vi "Dashboard Main.vi"() -> ()   [LabVIEW 2018]
uses:
  <vilib>/Utility/miscctls.llb/LVRowAndColumnTypeDef.ctl
  <vilib>/event_ctls.llb/eventvkey.ctl
  <vilib>/Rock Robotics/Network Tables/NT Read Numeric Array.vi
  <vilib>/Rock Robotics/WPI/Dashboard/WPI_DashboardLogging Global.vi
panel:
  in  "Camera Settings Right":T1={"Frame Rate"=30, "Compression"=30, "Size"=1, "DB Camera Config"=FALSE} {"Frame Rate" scale=1.0..30.0; "Compression" scale=100.0..-1.0; "Size" items=["640x480", "320x240", "160x120"]}
  in  "Camera Name Right":string(combo)="No Camera Selection"
  out "Camera Perf":string
  in  "Camera Settings":T1={"Frame Rate"=30, "Compression"=30, "Size"=1, "DB Camera Config"=FALSE} {"Frame Rate" scale=1.0..30.0; "Compression" scale=100.0..-1.0; "Size" items=["640x480", "320x240", "160x120"]}
  in  "TCP":refnum<k5>
  in  "Rec Mode":enum32{"Stop", "Record", "Playback"}(radio)
  out "Robot IP":string
  out "Image Message":string="Timeout in Camera Communications"
  in  "Dashboard Tab":T2(tab)
  out "Distance":dbl
  out "y2 (R)":dbl
  out "x2 (R)":dbl
  out "y1 (L)":dbl
  out "x1 (L)":dbl
  in  ".Avg Factor":i32=1
  in  "Enable Vision\nProcessing":bool
  in  "Reset":bool
  out "Total Stored\nSince Reset":i32
  in  "# New Images\nto Store":i32=1
  in  "Photo\nStore Rate":u32=100
  in  "Start\nStoring":bool
  in  "Select Auto":string(combo)="Select Autonomous ..."
  out "NT Connection":bool
  out "MotorChart R":cluster{"Numeric":dbl, "Numeric":dbl}(graph)
  out "MotorChart L":cluster{"Numeric":dbl, "Numeric":dbl}(graph)
  out "MotorSliders R":cluster{"MotorSlide1":dbl, "MotorSlide2":dbl} {"MotorSlide2" scale=-1.0..1.0 scale format="%#_2e"; "MotorSlide1" scale=-1.0..1.0 scale format="%#_2e"}
  out "MotorSliders L":cluster{"MotorSlide1":dbl, "MotorSlide2":dbl} {"MotorSlide2" scale=-1.0..1.0 scale format="%#_2e"; "MotorSlide1" scale=-1.0..1.0 scale format="%#_2e"}
  out "Gyro":dbl(knob) scale=0.0..360.0
  out "JS1 Z":dbl(slide) scale=-1.0..1.0 scale format="%#_2e"
  out "JS1 Graph":cluster{"X":dbl, "Y":dbl}[](graph)
  out "JS1 Buttons":T3
  out "JS2 Z":dbl(slide) scale=-1.0..1.0 scale format="%#_2e"
  out "JS2 Graph":cluster{"X":dbl, "Y":dbl}[](graph)
  out "JS2 Buttons":T3
  out "Mode":T4(ring)=enum."Auto Disabled"
  out "Right Camera Perf":cluster{"Bandwidth (Mbps)":dbl, "FPS":dbl}
  out "Camera Image Right":T5(plugin-control)
  in  "DB/String 9":string
  in  "DB/String 8":string
  in  "DB/String 7":string
  in  "DB/String 6":string
  in  "DB/String 5":string
  in  "DB/String 4":string
  in  "DB/String 3":string
  in  "DB/String 2":string
  in  "DB/String 1":string
  in  "DB/String 0":string
  in  "DB/Slider 0":dbl(slide) scale=0.0..5.0
  in  "DB/Slider 1":dbl(slide) scale=0.0..5.0
  in  "DB/Slider 2":dbl(slide) scale=0.0..5.0
  in  "DB/Slider 3":dbl(slide) scale=0.0..5.0
  out "DB/LED 3":bool
  out "DB/LED 2":bool
  out "DB/LED 1":bool
  out "DB/LED 0":bool
  in  "DB/Button 3":bool
  in  "DB/Button 2":bool
  in  "DB/Button 1":bool
  in  "DB/Button 0":bool caption="New Name"
  in  "Test Slider":dbl(slide) scale=0.0..100.0 scale format="%#_3g"
  in  "On/Off":bool caption="Solenoid"
  in  "Test Name":u16(ring) items=["Select the test to run..."]
  in  "Test Tree":string(tree)
  in  "Motor":cluster{"Value":dbl, "Enable":bool} {"Value" scale=-1.0..1.0 scale format="%#_3g"}
  out "Progress":T6 {"Test Progress" scale=0.0..100.0}
  in  "Rev/Fwd":cluster{"Forward":bool, "Reverse":bool}
  in  "Test Ring":u16(ring) items=["Monochrome", "Color"]
  out "Cmd Status":string
  in  "Execute Command":bool
  in  "Command Params":string[][](table)
  in  "Command Selection":i32(listbox)
  in  "CheckList":i32(listbox)
  out "Tree":string(tree)
  out "Camera Image":T5(plugin-control)
  out "Background":bool
  in  "Camera Name":string(combo)="No Camera Selection"
  # "HW"
  # "HW"
  # "Joysticks"
  # "Drive Motors"
  # "Front"
  # "Right"
  # "Left"
  # "Back"
  # "This tab is a great place for autonomous settings and robot-specific values.\nPlace controls and indicators inside this tab and match name to\nDashboard Variables on robot. You can also delete this comment."
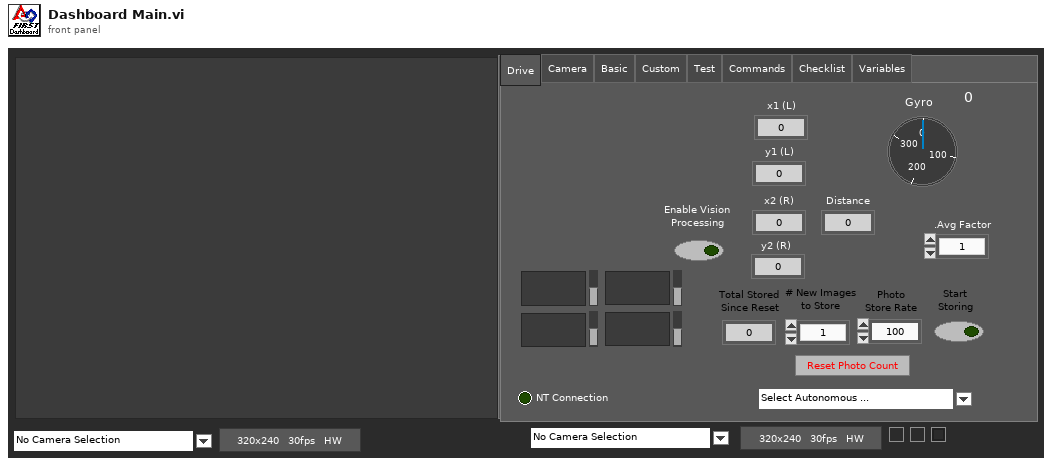
[diagram p1: front panel]
types:
  T1 = cluster{"Frame Rate":i32, "Compression":i32, "Size":u16, "DB Camera Config":bool}
  T2 = enum32{"Drive", "Camera", "Basic", "Custom", "Test", "Commands", "Checklist", "Variables"}
  T3 = cluster{bool, bool, bool, bool, bool, bool, bool, bool, bool, bool, bool, bool}
  T4 = enum8{"Tele-Op Disabled", "Tele-Op Enabled", "Auto Disabled", "Auto Enabled", "Test Disabled", "Test Enabled", "Disconnected", "No Code", "E-Stop"}
  T5 = typedef "IMAQ Image.ctl" = refnum<image>
  T6 = cluster{"Test Progress":u8, "Test Progress Text":string}
  T7 = cluster{"Save Path":path, "Interval (s)":dbl, "Keep":i32}
  T8 = typedef "Image Type" = u32
  T9 = cluster{"IDs":cluster{"RPC field ID":u16, "Unique ID":u16}, "String":string}
  T10 = cluster{"Camera Image":refnum<vi>, "Dashboard Tab":refnum<vi>, "Background":refnum<vi>, "Rec Mode":refnum<vi>, "Test Slider":refnum<vi>, "On/Off ":refnum<vi>, "Test Ring":refnum<vi>, "Rev/Fwd":refnum<vi>, "Test Name":refnum<vi>, "Motor":refnum<vi>, "Progress":refnum<vi>, "CheckList":refnum<vi>, "Tree":refnum<vi>, "Test Tree":refnum<vi>, "Command Params":refnum<vi>, "Command Selection":refnum<vi>, "Execute Command":refnum<vi>, "Cmd Status":refnum<vi>, "Camera Settings":refnum<vi>, "Camera Name":refnum<vi>, "Camera Perf":refnum<vi>, "Camera Settings Right":refnum<vi>, "Camera Name Right":refnum<vi>, "Camera Image Right":refnum<vi>}
  T11 = cluster{"Global Rectangle":i32[], "Contours":cluster{"Contour Type":u32, "ROI Type":u32, "Points":i32[]}[]}
  T12 = cluster{"Camera Name":string, string, "Saved DB Images Info":cluster{"Save Path":path, "Interval (s)":dbl, "Keep":i32}}
  T13 = cluster{"Pixels ":cluster{"Start":cluster{"X":dbl, "Y":dbl}, "End":cluster{"X":dbl, "Y":dbl}}, "Real World":cluster{"Start":cluster{"X":dbl, "Y":dbl}, "End":cluster{"X":dbl, "Y":dbl}}}
  T14 = cluster{"Start":cluster{"X":dbl, "Y":dbl}, "End":cluster{"X":dbl, "Y":dbl}}
  T15 = cluster{"Camera Name Right":string, string, "Saved DB Images Info":cluster{"Save Path":path, "Interval (s)":dbl, "Keep":i32}}
  T16 = cluster{"Error Strings":string, "Disable Counts":cluster{u16, u16}, "Rail Faults":cluster{u16, u16, u16}, "Robot IP":string, "DB Mode":u8, "Event Info":cluster{"Name":string, "Type":u8, "Number":u16, "Replay":u8}}
  T17 = cluster{"Storage":cluster{"Disk Free":u64, "RAM Block":u32, "RAM free":u32}, "CPU Utilization":cluster{"CPU % ISR":sgl, "CPU % Time Crit":sgl, "CPU % Timed Str":sgl, "CPU % High":sgl, "CPU % Above":sgl, "CPU % Normal":sgl, "CPU % Low":sgl}, "CAN":cluster{"% Bus Utilization":sgl, "Bus Off Cnt":u32, "TX_FIFO Full Cnt":u32, "Receive Error Cnt":u8, "Transmit Error Cnt":u8}, "HID":cluster{"HID Outputs":u32, "Rumble Low":u16, "Rumble High":u16}[]}
  T18 = cluster{"Status bits":cluster{"Test Mode":bool, "Autonomous":bool, "Enabled":bool, "Code Start":bool, "Brownout":bool, "Reserved 2":bool, "Reserved 3":bool, "E-Stop":bool}, "Code Trace":cluster{"Disabled":bool, "TeleOp":bool, "Auto":bool, "Test":bool}, "Controller Type":enum16{"unknown", "cRIO", "roboRio"}, "Code?":enum16{"unknown", "noCode", "code"}, "Battery V":dbl}
  T19 = cluster{"Control Bits":cluster{"TestMode":bool, "Autonomous":bool, "Enabled":bool, "FMS Present":bool, bool, bool, bool, "E-Stop":bool}, "Team Station ":u8, "Countdown":sgl, "Joystick Values":cluster{"Axes":dbl[], "Buttons":bool[], "POVs":i16[]}[]}
  T20 = cluster{"Axes":dbl[], "Buttons":bool[], "POVs":i16[]}[]
  T21 = cluster{"Axes":dbl[], "Buttons":bool[], "POVs":i16[]}
  T22 = cluster{"Buttons[0]":bool, "Buttons[1]":bool, "Buttons[2]":bool, "Buttons[3]":bool, "Buttons[4]":bool, "Buttons[5]":bool, "Buttons[6]":bool, "Buttons[7]":bool, "Buttons[8]":bool, "Buttons[9]":bool, "Buttons[10]":bool, "Buttons[11]":bool}
  T23 = cluster{"Operation":enum16{"Update", "Clear"}, "Color Box":u32}[]
  T24 = typedef "eventvkey.ctl" = enum16{"ASCII", "Enter", "Return", "Shift", "Ctrl", "Alt", "Cmd", "Opt", "Caps", "NumLock", "Clear", "Break", "Up", "Down", "Left", "Right", "Insert", "Delete", "Home", "End", "PageUp", "PageDown", "Escape", "Help", "Pause", "ScrollLock", "F1", "F2", "F3", "F4", "F5", "F6", "F7", "F8", "F9", "F10", "F11", "F12", "F13", "F14", "F15", "F16", "F17", "F18", "F19", "F20", "F21", "F22", "F23", "F24", "Play", "VolumeUp", "VolumeDown", "Mute", "Two Byte Char"}
  T25 = cluster{"Image Size":bool, "Image Type":bool, "Pixel Value":bool, "ROI Information":bool, "Zoom Factor":bool}
  T26 = cluster{"Operation":enum16{"Update", "Clear"}, "Color Box":u32}
  T27 = typedef "LVRowAndColumnTypeDef.ctl" = cluster{"Row":i32, "Column":i32}
  T28 = cluster{"Shift":bool, "Ctrl":bool, "Alt":bool, "Cmd":bool, "Opt":bool}
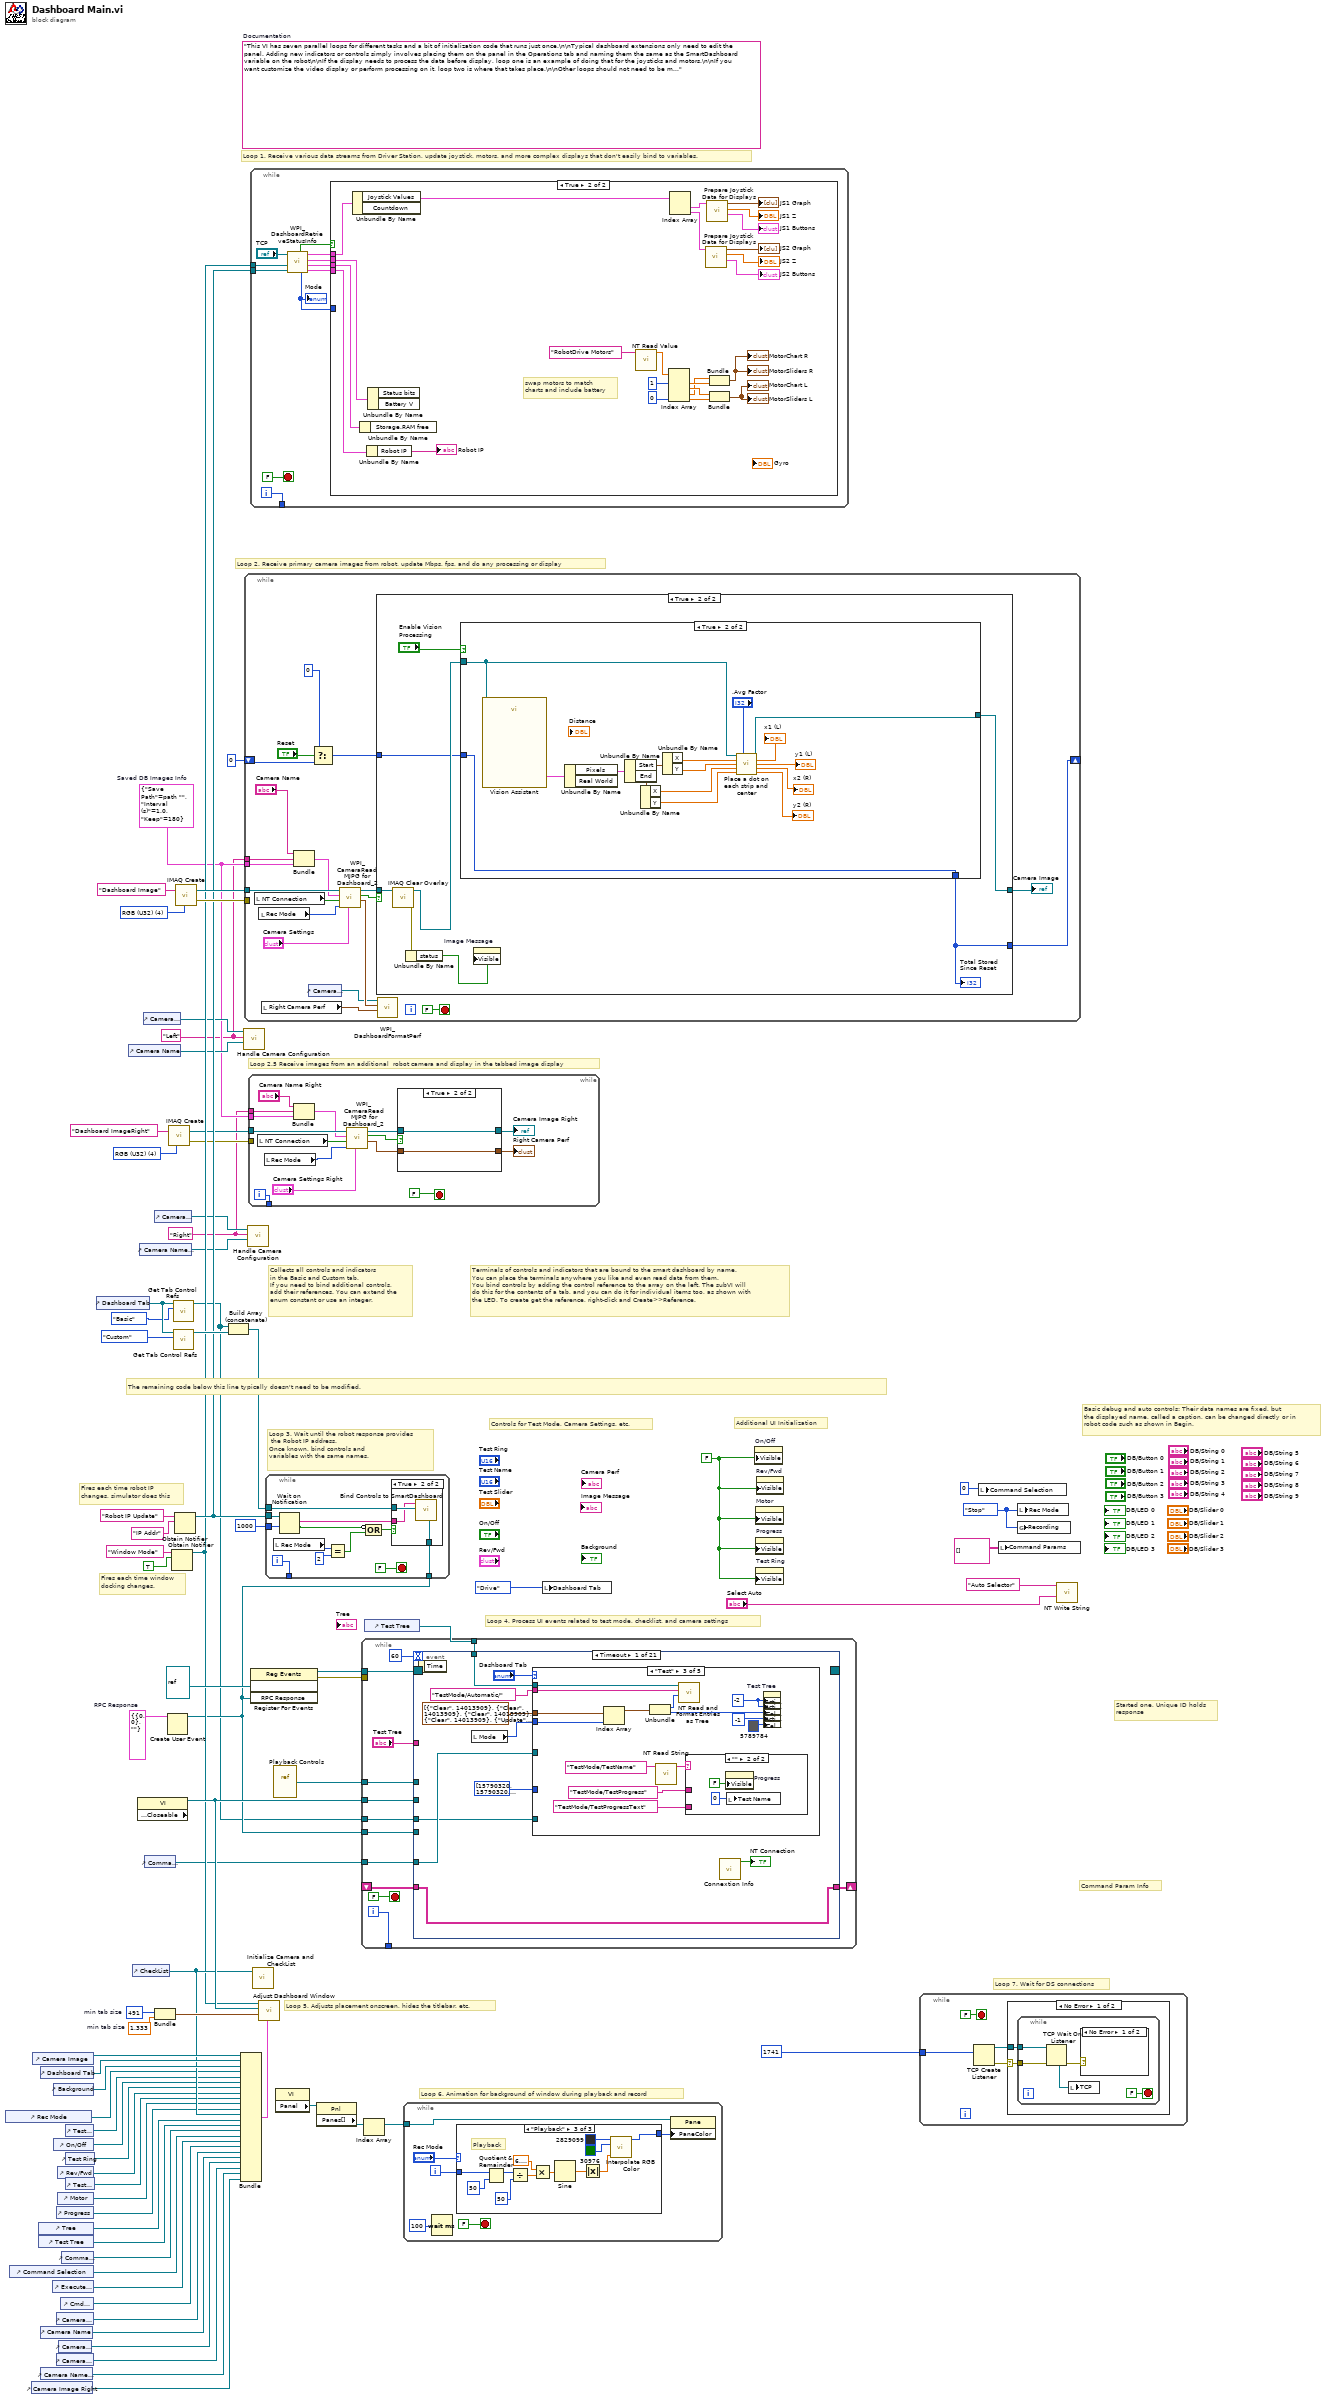
[diagram p0: block diagram]
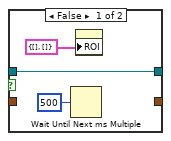
[diagram p2: hidden frame]
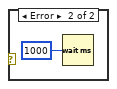
[diagram p3: hidden frame]
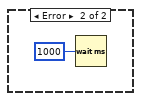
[diagram p4: hidden frame]
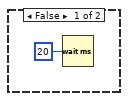
[diagram p5: hidden frame]
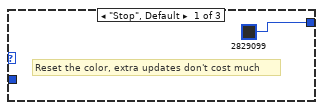
[diagram p6: hidden frame]
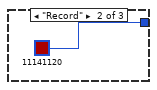
[diagram p7: hidden frame]
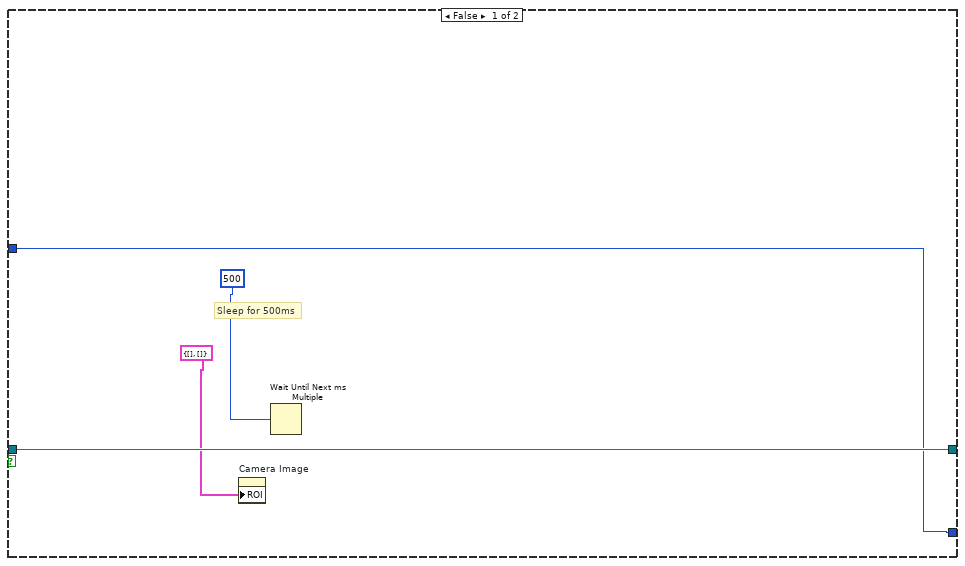
[diagram p9: hidden frame]
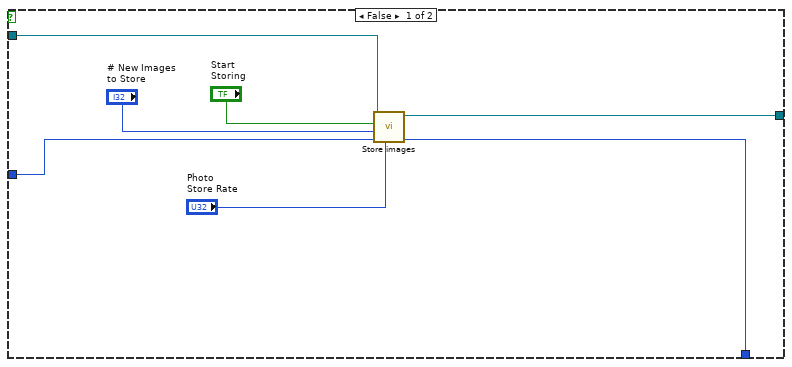
[diagram p10: hidden frame]
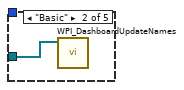
[diagram p12: hidden frame]
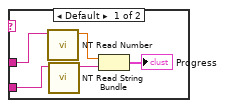
[diagram p13: hidden frame]
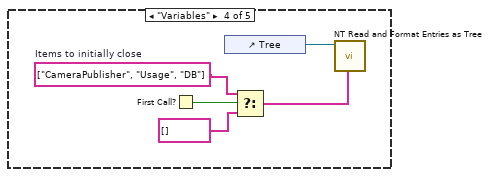
[diagram p14: hidden frame]
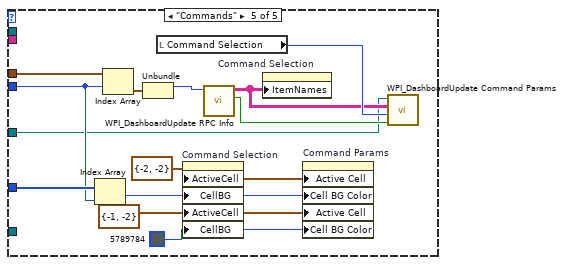
[diagram p15: hidden frame]
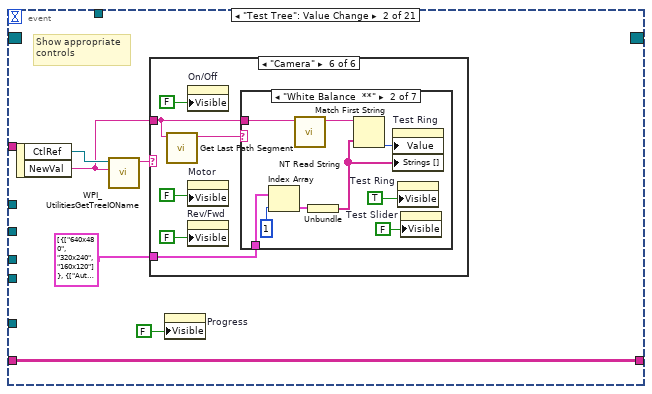
[diagram p16: hidden frame]
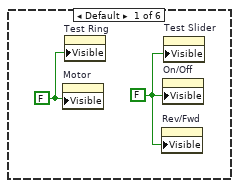
[diagram p17: hidden frame]
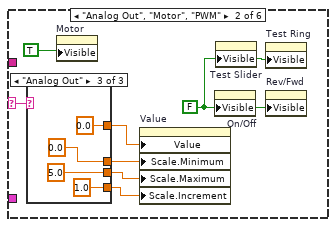
[diagram p18: hidden frame]
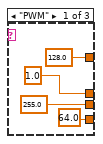
[diagram p19: hidden frame]
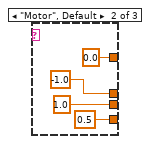
[diagram p20: hidden frame]
diagram:
  w4 = T7 {"Save Path"=path "", "Interval (s)"=1.0, "Keep"=180}  # Saved DB Images Info
  w3 = "Right"
  w2 = "Left"
  w14 = T8 4 items=["Grayscale (U8)", "Grayscale (I16)", "Grayscale (SGL)", "Complex (CSG)", "RGB (U32)", "HSL (U32)", "RGB (U64)"] ("Image Type")
  w30 = T9 {"IDs"={"RPC field ID"=0, "Unique ID"=0}, "String"=""}  # RPC Response
  w53 = 491  # min tab size
  w52 = 1.333  # min tab size
  w60 = enum32{"Stop", "Record", "Playback"}."Stop" ("Rec Mode")
  w37 = FALSE ("Visible")
  (unwired) "This VI has seven parallel loops for different tasks and a bit of initialization code that runs just once.\n\nTypical dashboard extensions only need to edit the panel. Adding new indicators or controls simply involves placing them on the panel in the Operations tab and naming them the same as the SmartDashboard variable on the robot\n\nIf the display needs to process the data before display, loop one is an example of doing that for the joysticks and motors.\n\nIf you want customize the video display or perform processing on it, loop two is where that takes place.\n\nOther loops should not need to be modified. They are pretty standard, and document the task they perform."  # Documentation
  w77 = T8 4 items=["Grayscale (U8)", "Grayscale (I16)", "Grayscale (SGL)", "Complex (CSG)", "RGB (U32)", "HSL (U32)", "RGB (U64)"] ("Image Type")
  # "Loop 2.5 Receive images from an additional  robot camera and display in the tabbed image display"
  # "Command Param Info"
  # "Started one, Unique ID holds\nresponse"
  # "Loop 7. Wait for DS connections"
  # "Basic debug and auto controls: Their data names are fixed, but\nthe displayed name, called a caption, can be changed directly or in\nrobot code such as shown in Begin."
  # "Controls for Test Mode, Camera Settings, etc."
  # "Additional UI Initialization"
  # "Loop 6. Animation for background of window during playback and record"
  # "Fires each time robot IP\nchanges, simulator does this"
  # "Fires each time window\ndocking changes."
  # "Collects all controls and indicators\nin the Basic and Custom tab.\nIf you need to bind additional controls,\nadd their references. You can extend the\nenum constant or use an integer."
  # "The remaining code below this line typically doesn't need to be modified."
  # "Loop 4. Process UI events related to test mode, checklist, and camera settings"
  # "Terminals of controls and indicators that are bound to the smart dashboard by name.\nYou can place the terminals anywhere you like and even read data from them.\nYou bind controls by adding the control reference to the array on the left. The subVI will\ndo this for the contents of a tab, and you can do it for individual items too, as shown with\nthe LED. To create get the reference, right-click and Create>>Reference."
  # "Loop 3. Wait until the robot response provides\n the Robot IP address.\nOnce known, bind controls and\nvariables with the same names."
  # "Loop 5. Adjusts placement onscreen, hides the titlebar, etc."
  # "Loop 1. Receive various data streams from Driver Station, update joystick, motors, and more complex displays that don't easily bind to variables."
  # "Loop 2. Receive primary camera images from robot, update Mbps, fps, and do any processing or display"
  n1 = control-ref of="Rec Mode"() -> (w43:refnum<vi>)
  n2 = control-ref of="Command Selection"() -> (w29:refnum<vi>)
  n3 = control-ref of="Camera Image Right"() -> (w7:refnum<vi>)
  n4 = control-ref of="Camera Image"() -> (w55:refnum<vi>)
  n5 = control-ref of="Tree"() -> (w47:refnum<vi>)
  n6 = control-ref of="Test Tree"() -> (w46:refnum<vi>)
  n7 = control-ref of="Dashboard Tab"() -> (w54:refnum<vi>)
  n8 = control-ref of="Camera Name"() -> (w20:refnum<vi>)
  n9 = control-ref of="Camera Name Right"() -> (w8:refnum<vi>)
  n10 = control-ref of="Execute Command"() -> (w31:refnum<vi>)
  n11 = control-ref of="Background"() -> (w50:refnum<vi>)
  n12 = control-ref of="On/Off"() -> (w41:refnum<vi>)
  n13 = control-ref of="Progress"() -> (w38:refnum<vi>)
  n14 = control-ref of="Camera Settings"() -> (w21:refnum<vi>)
  n15 = control-ref of="Camera Settings Right"() -> (w9:refnum<vi>)
  n16 = control-ref of="Rev/Fwd"() -> (w39:refnum<vi>)
  n17 = control-ref of="Motor"() -> (w44:refnum<vi>)
  n18 = control-ref of="Camera Perf"() -> (w19:refnum<vi>)
  n19 = control-ref of="Cmd Status"() -> (w25:refnum<vi>)
  n20 = control-ref of="Command Params"() -> (w32:refnum<vi>)
  n21 = control-ref of="Test Slider"() -> (w42:refnum<vi>)
  n22 = control-ref of="Test Ring"() -> (w40:refnum<vi>)
  n23 = control-ref of="Test Name"() -> (w45:refnum<vi>)
  n24 = control-ref of="Dashboard Tab"() -> (w58:refnum<vi>)
  n25 = control-ref of="Camera Name"() -> (w22:refnum<vi>)
  n26 = control-ref of="CheckList"() -> (w48:refnum<vi>)
  n27 = property class="VI" props=["Front Panel.Closeable"]() -> (reference out=w59:refnum<vi>)  [unwired: 2 in, 2 out]
  n28 = control-ref of="Camera Name Right"() -> (w10:refnum<vi>)
  n29 = control-ref of="Camera Settings"() -> (w23:refnum<vi>)
  n30 = control-ref of="Command Params"() -> (w24:refnum<vi>)
  n31 = control-ref of="Camera Settings Right"() -> (w11:refnum<vi>)
  n32 = Bundle("min tab size"=w53, "min tab size"=w52) -> (w51:cluster{"min tab size":i32, "min tab size":dbl})  [unwired: 1 in]
  n33 = Create User Event(user event datatype=w30) -> (user event=w26:refnum<user-event>)  [unwired: 1 in, 1 out]
  n34 = call "IMAQ Create"("Image Name"="Dashboard ImageRight", "Image Type"=w14) -> ("New Image"=w13:T5, "error out"=w12:errorcluster)  [unwired: 2 in, 1 out]
  n35 = Obtain Notifier(name (unnamed)="Window Mode", notification data type=TRUE) -> (notifier out=w35:refnum<notifier>)  [unwired: 2 in, 2 out]
  n36 = call <vilib>:"Get Tab Control Refs.vi"("Page Index"=T2."Basic" ("Dashboard Tab"), "TabControl in"=w58) -> ("ControlsOnPage"=w18:refnum<vi>[])  [unwired: 9 in]
  n37 = call <vilib>:"Get Tab Control Refs.vi"("Page Index"=T2."Custom" ("Dashboard Tab"), "TabControl in"=w58) -> ("ControlsOnPage"=w57:refnum<vi>[])  [unwired: 9 in]
  n38 = Obtain Notifier(name (unnamed)="Robot IP Update", notification data type="IP Addr" ("name (unnamed)")) -> (notifier out=w36:refnum<notifier>)  [unwired: 2 in, 2 out]
  n39 = call "IMAQ Create"("Image Name"="Dashboard Image", "Image Type"=w77) -> ("New Image"=w75:T5, "error out"=w74:errorcluster)  [unwired: 2 in, 1 out]
  n40 = Build Array (concatenate)(w18, w57) -> (w56:refnum<vi>[])
  n41 = Bundle("Camera Image"=w55, "Dashboard Tab"=w54, "Background"=w50, "Rec Mode"=w43, "Test Slider"=w42, "On/Off"=w41, "Test Ring"=w40, "Rev/Fwd"=w39, "Test Name"=w45, "Motor"=w44, "Progress"=w38, "CheckList"=w48, "Tree"=w47, "Test Tree"=w46, "Command Params"=w32, "Command Selection"=w29, "Execute Command"=w31, "Cmd Status"=w25, "Camera Settings"=w21, "Camera Name"=w20, "Camera Perf"=w19, "Camera Settings Right"=w9, "Camera Name Right"=w8, "Camera Image Right"=w7) -> (w49:T10)  [unwired: 1 in]
  n42 = call "Handle Camera Configuration.vi"("CameraNameRef"=w22, "Display Name"=w2, "ClusterRef"=w23) -> ()  [unwired: 9 in]
  n43 = while {
    tunnel: w75 -> [w96]
    tunnel: w74 -> [_]
    tunnel: w4 -> [w89]
    tunnel: w2 -> [w86]
    shift-right: [w78] -> _
    shift-left: 0 -> [w81]
    stop <- FALSE stop-if-true
    n44 = local read "NT Connection"() -> (w90:bool)
    n45 = local read "Rec Mode"() -> (w93:enum32{"Stop", "Record", "Playback"})
    n46 = local read "Right Camera Perf"() -> (w84:cluster{"Bandwidth (Mbps)":dbl, "FPS":dbl})
    n47 = Bundle("Camera Name"="Camera Name", w86, "Saved DB Images Info"=w89) -> (w88:T12)  [unwired: 1 in]
    n48 = control-ref of="Camera Perf"() -> (w83:refnum<vi>)
    n49 = Select(t=0, s="Reset", f=w81) -> (s? t:f=w79:i32)
    n50 = call <vilib>:"WPI_CameraRead MJPG for Dashboard_2.vi"("Camera Settings"="Camera Settings", "Rec Mode"=w93, "NT Connection"=w90, "Capture Info"=w88, "Image in"=w96) -> ("perf info"=w85:cluster{"Bandwidth (Mbps)":dbl, "fps":dbl}, "Active"=w94:bool, "Image\\ out"=w95:T5)  [unwired: 4 in]
    n51 = case shown="True" w94 {
      tunnel: w95 -> [w100 w107]
      tunnel: [w100 w103] -> w91
      tunnel: w79 -> [w98 w104]
      tunnel: [w98 w102] -> w78
      frame False {
        # "Sleep for 500ms"
        n52 = property on="Camera Image" class="ImageControl"("ROI"=T11 {"Global Rectangle"=[], "Contours"=[]}) -> ()  [unwired: 2 in, 2 out]
        n53 = Wait Until Next ms Multiple(millisecond multiple=u32 500) -> ()  [unwired: 1 out]
      }
      frame True {
        n54 = call "IMAQ Clear Overlay"("Image"=w107) -> ("error out"=w108:errorcluster, "Image Out"=w105:T5)  [unwired: 2 in, 7 out]
        n55 = Unbundle By Name(w108) -> ("status"=w109:bool)
        n56 = case shown="True" "Enable Vision\nProcessing" {
          tunnel: w105 -> [w113 w124]
          tunnel: w104 -> [w112 w130]
          tunnel: [w111 w123] -> w103
          tunnel: [w110 w130] -> w102
          frame False {
            n57 = call "Store images.vi"("ms Capture Rate"="Photo\nStore Rate", "# Total images IN"=w112, "# new images to capture"="# New Images\nto Store", "Store # Images?"="Start\nStoring", "Image"=w113) -> ("Total images OUT"=w110:i32, "Image Out"=w111:T5)  [unwired: 5 in]
          }
          frame True {
            n58 = call "Vision Assistant"("Image In"=w124) -> ("Clamp Points (Max Clamp 1)"=w132:T13)  [unwired: 23 in, 3 out]
            n59 = Unbundle By Name(w132) -> ("Pixels"=w131:T14)  [unwired: 1 out]
            n60 = Unbundle By Name(w131) -> ("Start"=w129:cluster{"X":dbl, "Y":dbl}, "End"=w128:cluster{"X":dbl, "Y":dbl})
            n61 = Unbundle By Name(w128) -> ("X"=w118:dbl, "Y"=w117:dbl)
            n62 = Unbundle By Name(w129) -> ("X"=w127:dbl, "Y"=w126:dbl)
            n63 = call "Place a dot on each strip and center.vi"("Image"=w124, "Avg Factor"=".Avg Factor", "x1 (L) IN"=w127, "y1 (L) IN"=w126, "x2 (R) IN"=w118, "y2 (R) IN"=w117) -> ("Image Out"=w123:T5, "x1 (L) out"=→"x1 (L)":dbl, "y1 (L) out"=→"y1 (L)":dbl, "x2 (R) out"=→"x2 (R)":dbl, "y2 (R) out"=→"y2 (R)":dbl)  [unwired: 5 in]
          }
        }
        "Total Stored\nSince Reset" <- w102
        n64 = property on="Image Message" class="Str"("Visible"=w109) -> ()  [unwired: 2 in, 2 out]
      }
    }
    "Camera Image" <- w91
    n65 = call <vilib>:"WPI_DashboardFormatPerf.vi"("Right Camera Perf"=w84, "Performance"=w85, "String in"=w83) -> ()  [unwired: 9 in]
  }
  n66 = call "Handle Camera Configuration.vi"("CameraNameRef"=w10, "Display Name"=w3, "ClusterRef"=w11) -> ()  [unwired: 9 in]
  n67 = while {
    tunnel: w13 -> [w147]
    tunnel: w12 -> [_]
    tunnel: [w142] -> _
    tunnel: w4 -> [w138]
    tunnel: w3 -> [w135]
    i -> [w142]
    stop <- FALSE stop-if-true
    n68 = local read "NT Connection"() -> (w139:bool)
    n69 = local read "Rec Mode"() -> (w146:enum32{"Stop", "Record", "Playback"})
    n70 = Bundle("Camera Name Right"="Camera Name Right", w135, "Saved DB Images Info"=w138) -> (w137:T15)  [unwired: 1 in]
    n71 = call <vilib>:"WPI_CameraRead MJPG for Dashboard_2.vi"("Camera Settings"="Camera Settings Right", "Rec Mode"=w146, "NT Connection"=w139, "Capture Info"=w137, "Image in"=w147) -> ("perf info"=w133:cluster{"Bandwidth (Mbps)":dbl, "fps":dbl}, "Active"=w141:bool, "Image\\ out"=w144:T5)  [unwired: 4 in]
    n72 = case shown="True" w141 {
      tunnel: w144 -> [w149 w152]
      tunnel: [w149 w152] -> w140
      tunnel: [_ w151] -> w134
      tunnel: w133 -> [_ w151]
      frame False {
        n73 = Wait Until Next ms Multiple(millisecond multiple=u32 500) -> ()  [unwired: 1 out]
        n74 = property on="Camera Image Right" class="ImageControl"("ROI"=T11 {"Global Rectangle"=[], "Contours"=[]}) -> ()  [unwired: 2 in, 2 out]
      }
      frame True {
      }
    }
    "Camera Image Right" <- w140
    "Right Camera Perf" <- w134
  }
  n75 = while {
    tunnel: [w162] -> _
    tunnel: w36 -> [w156]
    tunnel: w35 -> [w153]
    i -> [w162]
    stop <- FALSE stop-if-true
    n76 = call <vilib>:"WPI_DashboardRetrieveStatusInfo.vi"("Binding Refnum"=w156, "Window Mode Notifier"=w153, "TCP Cnx"="TCP") -> ("Power and Errors"=w157:T16, "Robot Metrics"=w160:T17, "Status Info"=w161:T18, "Control Info"=w158:T19, "Robot Mode"=w155:T4, "Process?"=w159:bool)  [unwired: 3 in]
    "Mode" <- w155
    n77 = case shown="True" w159 {
      tunnel: w161 -> [_ w188]
      tunnel: w160 -> [_ w187]
      tunnel: w158 -> [_ w186]
      tunnel: w157 -> [_ w185]
      tunnel: w155 -> [_ _]
      frame False {
        n78 = Wait (ms)(milliseconds to wait=u32 20) -> ()  [unwired: 1 out]
      }
      frame True {
        # "swap motors to match\ncharts and include battery"
        n79 = Unbundle By Name(w186) -> ("Joystick Values"=w176:T20)  [unwired: 1 out]
        n80 = Unbundle By Name(w187) -> ()  [unwired: 1 out]
        n81 = Unbundle By Name(w185) -> ("Robot IP"=→"Robot IP":string)
        n82 = Unbundle By Name(w188) -> ()  [unwired: 2 out]
        n83 = call-poly <vilib>:"NT Read Value.vi"("Name"="RobotDrive Motors") -> ("Numeric Array"=w166:dbl[])  [unwired: 9 in, 1 out]
        n84 = Index Array(array=w166, index #1=1, index #4=0) -> (element #1=w180:dbl, element #2=w181:dbl, element #3=w179:dbl, element #4=w184:dbl)  [unwired: 2 in]
        n85 = Index Array(array=w176) -> (element #1=w175:T21, element #2=w171:T21)  [unwired: 2 in]
        n86 = call "Prepare Joystick Data for Displays.vi"("Joystick Values"=w171) -> ("Buttons"=→"JS2 Buttons":T22, "Z Axis"=→"JS2 Z":dbl, "Cartesian Data"=→"JS2 Graph":cluster{"X axis":dbl, "X axis":dbl}[])  [unwired: 8 in]
        n87 = call "Prepare Joystick Data for Displays.vi"("Joystick Values"=w175) -> ("Buttons"=→"JS1 Buttons":T22, "Z Axis"=→"JS1 Z":dbl, "Cartesian Data"=→"JS1 Graph":cluster{"X axis":dbl, "X axis":dbl}[])  [unwired: 8 in]
        n88 = Bundle("Numeric"=w179, "Numeric"=w180) -> (→"MotorChart R" →"MotorSliders R":cluster{"Numeric":dbl, "Numeric":dbl})  [unwired: 1 in]
        n89 = Bundle("Numeric"=w181, "Numeric"=w184) -> (→"MotorChart L" →"MotorSliders L":cluster{"Numeric":dbl, "Numeric":dbl})  [unwired: 1 in]
      }
    }
  }
  n90 = register-events(refnum<vi> refnum, w26) -> (reference out=w64:refnum<event-registration>, error out=w63:errorcluster)  [unwired: 2 in]
  n91 = call "Initialize Camera and CheckList.vi"("ListBox in"=w48) -> ()  [unwired: 11 in]
  n92 = call "Adjust Dashboard Window.vi"("Sizing Refnums"=w49, "Size Constraints"=w51, "VI"=w59, "WIn Mode"=w35) -> ()  [unwired: 8 in]
  n93 = while {
    tunnel: w56 -> [w200]
    tunnel: w36 -> [w198]
    tunnel: [w196] -> _
    tunnel: u32 1000 ("milliseconds to wait") -> [w195]
    tunnel: w26 -> [w189]
    i -> [w196]
    stop <- FALSE stop-if-true
    n94 = local read "Rec Mode"() -> (w191:enum32{"Stop", "Record", "Playback"})
    n95 = Wait on Notification(notifier=w198, timeout in ms (-1)=w195) -> (notification=w197:string, timed out?=w193:bool)  [unwired: 2 in, 2 out]
    n96 = Equal?(x=w191, y=u16 2 ("Rec Mode")) -> (x = y?=w192:bool)
    n97 = Compound Arithmetic op=OR(invert w193, w192) -> (w194:bool)
    n98 = case shown="True" w194 {
      tunnel: w200 -> [_ w203]
      tunnel: w197 -> [_ w202]
      tunnel: w189 -> [_ w201]
      frame False {
      }
      frame True {
        n99 = call <vilib>:"Bind Controls to SmartDashboard.vi"("RPC ref"=w201, "Bound Control Refs"=w203, "Server IP Address"=w202) -> ()  [unwired: 9 in]
      }
    }
  }
  n100 = vi-ref "Playback Controls.vi"() -> (w65:refnum<vi>)
  n101 = property class="VI"() -> ("Panel"=w67:refnum<vi>)  [unwired: 2 in, 2 out]
  n102 = property class="Pnl"(reference=w67) -> ("Panes[]"=w68:refnum<vi>[])  [unwired: 1 in, 2 out]
  n103 = Index Array(array=w68) -> (element=w66:refnum<vi>)  [unwired: 1 in]
  n104 = control-ref of="Test Tree"() -> (w69:refnum<vi>)
  n105 = while {
    tunnel: [w213] -> _
    tunnel: w69 -> [w212]
    tunnel: w65 -> [w211]
    tunnel: w64 -> [w210]
    tunnel: w63 -> [_]
    tunnel: w59 -> [w209]
    tunnel: w26 -> [w208]
    tunnel: w24 -> [w207]
    shift-right: [w206] -> _
    shift-left: _ -> [w205]
    tunnel: w18 -> [w204]
    i -> [w213]
    stop <- FALSE stop-if-true
    n106 = event shown="[0] Timeout" {
      selector: w210 -> [_ _ _ _ _ _ _ _ _ _ _ _ _ _ _ _ _ _ _ _ _]
      dyn-events: [_ _ _ _ _ _ _ _ _ _ _ _ _ _ _ _ w473 _ _ _ _] -> _
      timeout: u32 60 ("milliseconds to wait") -> [_ _ _ _ _ _ _ _ _ _ _ _ _ _ _ _ _ _ _ _ _]
      tunnel: w212 -> [w225 _ _ _ _ _ _ _ _ _ _ _ _ _ _ _ _ _ _ _ _]
      tunnel: "Test Tree" -> [_ _ _ _ _ _ _ _ _ _ _ w440 w448 w450 w454 w462 _ _ _ _ _]
      tunnel: w211 -> [_ _ _ _ _ _ _ _ _ _ _ _ _ _ _ _ w475 _ w493 _ _]
      tunnel: w209 -> [_ _ _ _ _ _ _ _ _ _ _ _ _ _ _ _ w471 _ _ _ _]
      tunnel: w208 -> [_ _ _ _ _ _ _ _ _ _ _ _ _ _ _ _ w469 _ _ _ _]
      tunnel: w207 -> [w220 _ _ _ _ _ w391 _ _ _ _ _ _ _ _ _ _ _ _ _ _]
      tunnel: [w219 w268 w370 w375 w384 w388 w389 w398 w408 w415 w427 w439 w446 w449 w453 w461 w468 w488 w490 w494 w507] -> w206
      tunnel: w205 -> [w219 w268 w370 w375 w384 w388 w389 _ _ w415 w427 w439 w446 w449 w453 w461 w468 w488 w490 w494 w507]
      tunnel: w204 -> [w217 _ _ _ _ _ _ _ _ _ _ _ _ _ _ _ _ _ _ _ _]
      event Timeout {
        n107 = event-data() -> ()  [unwired: 1 in, 1 out]
        n108 = local read "Mode"() -> (w222:T4)
        n109 = case shown="\"Test\"" "Dashboard Tab" {
          tunnel: w225 -> [_ _ w241 _ _]
          tunnel: "TestMode/Automatic/" ("Name Pattern") -> [_ _ w240 _ _]
          tunnel: T23 [{"Operation"=enum."Clear", "Color Box"=14013909}, {"Operation"=enum."Clear", "Color Box"=14013909}, {"Operation"=enum."Clear", "Color Box"=14013909}, {"Operation"=enum."Clear", "Color Box"=14013909}, {"Operation"=enum."Update", "Color Box"=14013909}, {"Operation"=enum."Update", "Color Box"=16777215}, {"Operation"=enum."Clear", "Color Box"=14013909}, {"Operation"=enum."Clear", "Color Box"=14013909}, {"Operation"=enum."Clear", "Color Box"=14013909}] -> [_ _ w233 _ w261]
          tunnel: w222 -> [_ _ w232 _ w260]
          tunnel: u32[] [15790320, 15790320, 15790320, 15790320, 16777215, 16777215, 15790320, 15790320, 15790320] -> [_ _ _ _ w266]
          tunnel: w220 -> [_ _ _ _ w254]
          tunnel: w217 -> [_ w227 _ _ _]
          frame "Custom", Default {
          }
          frame "Basic" {
            n110 = call <vilib>:"WPI_DashboardUpdateNames.vi"("Controls on Tab"=w227) -> ()  [unwired: 11 in]
          }
          frame "Test" {
            w239 = -2 ("Active Item:Row Number")
            n111 = Index Array(array=w233, index=w232) -> (element=w234:T26)
            n112 = Unbundle(w234) -> ("Operation"=w235:enum16{"Update", "Clear"}, "Color Box"=w236:u32)
            n113 = call <vilib>:"NT Read String.vi"("Name"="TestMode/TestName") -> ("String"=w230:string)  [unwired: 9 in, 1 out]
            n114 = call <vilib>:"NT Read and Format Entries as Tree.vi"("Operation"=w235, "Name Pattern"=w240, "Tree Refnum"=w241) -> ()  [unwired: 7 in, 2 out]
            n115 = case shown="\"\"" w230 {
              tunnel: "TestMode/TestProgress" ("Name") -> [w243 _]
              tunnel: "TestMode/TestProgressText" ("Name") -> [w242 _]
              frame Default {
                n116 = call <vilib>:"NT Read Number.vi"("Name"=w243) -> ("Numeric"=w244:dbl)  [unwired: 9 in, 1 out]
                n117 = call <vilib>:"NT Read String.vi"("Name"=w242) -> ("String"=w245:string)  [unwired: 9 in, 1 out]
                n118 = Bundle("Numeric"=w244, "String"=w245) -> (→"Progress":cluster{"Numeric":dbl, "String":string})  [unwired: 1 in]
              }
              frame "" {
                n119 = property on="Progress" class="Clust (strict)"("Visible"=FALSE) -> ()  [unwired: 2 in, 2 out]
                n120 = local write "Test Name"(u16 0) -> ()
              }
            }
            n121 = property on="Test Tree" class="Tree (strict)"("Active Item Row Number"=w239, "ActiveColNum"=w239, "CellBG"=w236, "Active Item Row Number"=-1 ("Active Item:Row Number"), "CellBG"=u32 5789784 ("Color Box")) -> ()  [unwired: 2 in, 2 out]
          }
          frame "Variables" {
            w251 = string[] ["CameraPublisher", "Usage", "DB"]  # Items to initially close
            n122 = First Call?() -> (First Call?: T/F=w252:bool)
            n123 = control-ref of="Tree"() -> (w253:refnum<vi>)
            n124 = Select(t=w251, s=w252, f=string[] []) -> (s? t:f=w249:string[])
            n125 = call <vilib>:"NT Read and Format Entries as Tree.vi"("Tags to  Close"=w249, "Tree Refnum"=w253) -> ()  [unwired: 8 in, 2 out]
          }
          frame "Commands" {
            w262 = u32 5789784 ("Color Box")
            w263 = T27 {"Row"=-1, "Column"=-2} ("Active Cell:Active Cell")
            w265 = T27 {"Row"=-2, "Column"=-2} ("Active Cell:Active Cell")
            n126 = Index Array(array=w266, index=w260) -> (element=w264:u32)
            n127 = Index Array(array=w261, index=w260) -> (element=w259:T26)
            n128 = Unbundle(w259) -> ("Operation"=w258:enum16{"Update", "Clear"})  [unwired: 1 out]
            n129 = local read "Command Selection"() -> (w257:i32)
            n130 = property on="Command Selection" class="MCListbox (strict)"("ActiveCell"=w265, "CellBG"=w264, "ActiveCell"=w263, "CellBG"=w262) -> ()  [unwired: 2 in, 2 out]
            n131 = call <vilib>:"WPI_DashboardUpdate RPC Info.vi"("Operation"=w258) -> ("update"=w256:bool, "commands"=w255:string[][])  [unwired: 9 in]
            n132 = property on="Command Selection" class="MCListbox (strict)"("ItemNames"=w255) -> ()  [unwired: 2 in, 2 out]
            n133 = property on="Command Params" class="Tbl (strict)"("Active Cell"=w265, "Cell BG Color"=w264, "Active Cell"=w263, "Cell BG Color"=w262) -> ()  [unwired: 2 in, 2 out]
            n134 = call <vilib>:"WPI_DashboardUpdate Command Params.vi"("Update"=w256, "NewVal"=w257, "Commands"=w255, "Param Tbl"=w254) -> ()  [unwired: 7 in, 1 out]
          }
        }
        n135 = call <vilib>:"Connextion Info.vi"() -> ("Connected"=→"NT Connection":bool)  [unwired: 10 in, 1 out]
      }
      event "Test Tree": Value Change {
        # "Show appropriate\ncontrols"
        n136 = event-data() -> ("CtlRef"=w271:refnum<vi>, "NewVal"=w269:string)  [unwired: 1 in]
        n137 = call <vilib>:"WPI_UtilitiesGetTreeIOName.vi"("NewVal"=w269, "TreeControl in"=w271) -> ("I/O Name"=w272:string)  [unwired: 9 in]
        n138 = case shown="\"Camera\"" w272 {
          selector: w272 -> [_ w279 _ w301 w310 _]
          tunnel: w269 -> [_ _ w298 w300 _ w317]
          tunnel: cluster{string[]}[] [{["640x480", "320x240", "160x120"]}, {["Auto", "Fixed indoor", "Fixed outdoor 1", "Fixed outdoor 2", "Fixed fluorescent 1", "Fixed fluorescent 2", "Hold current"]}, {["Auto", "Flicker-free 50 Hz", "Flicker-free 60 Hz", "Hold current"]}, {["None", "Prioritize frame rate", "Prioritize image quality"]}, {["Monochrome", "Color"]}] -> [_ _ _ _ _ w316]
          frame Default {
            w274 = FALSE ("Visible")
            w273 = FALSE ("Visible")
            n139 = property on="Motor" class="Clust (strict)"("Visible"=w273) -> ()  [unwired: 2 in, 2 out]
            n140 = property on="Test Ring" class="Ring (strict)"("Visible"=w273) -> ()  [unwired: 2 in, 2 out]
            n141 = property on="Rev/Fwd" class="Clust (strict)"("Visible"=w274) -> ()  [unwired: 2 in, 2 out]
            n142 = property on="On/Off" class="Bool (strict)"("Visible"=w274) -> ()  [unwired: 2 in, 2 out]
            n143 = property on="Test Slider" class="Slide (strict)"("Visible"=w274) -> ()  [unwired: 2 in, 2 out]
          }
          frame "Analog Out", "Motor", "PWM" {
            w280 = FALSE ("Visible")
            n144 = case shown="\"Analog Out\"" w279 {
              tunnel: [1.0 ("Value") -1.0 ("Value") 0.0 ("Value")] -> w278
              tunnel: [255.0 ("Value") 1.0 ("Value") 5.0 ("Value")] -> w277
              tunnel: [128.0 ("Value") 0.0 ("Value") 0.0 ("Value")] -> w276
              tunnel: [64.0 ("Value") 0.5 ("Value") 1.0 ("Value")] -> w275
              frame "PWM" {
              }
              frame "Motor", Default {
              }
              frame "Analog Out" {
              }
            }
            n145 = property on="Motor" class="Clust (strict)"("Visible"=TRUE) -> ()  [unwired: 2 in, 2 out]
            n146 = property on="Value" class="Slide (strict)"("Value"=w276, "Scale.Minimum"=w278, "Scale.Maximum"=w277, "Scale.Increment"=w275) -> ()  [unwired: 2 in, 2 out]
            n147 = property on="On/Off" class="Bool (strict)"("Visible"=w280) -> ()  [unwired: 2 in, 2 out]
            n148 = property on="Test Slider" class="Slide (strict)"("Visible"=w280) -> ()  [unwired: 2 in, 2 out]
            n149 = property on="Test Ring" class="Ring (strict)"("Visible"=w280) -> ()  [unwired: 2 in, 2 out]
            n150 = property on="Rev/Fwd" class="Clust (strict)"("Visible"=w280) -> ()  [unwired: 2 in, 2 out]
          }
          frame "Servo" {
            w296 = FALSE ("Visible")
            n151 = call <vilib>:"NT Read Number.vi"("Name"=w298) -> ("Numeric"=w297:dbl)  [unwired: 9 in, 1 out]
            n152 = property on="Test Slider" class="Slide (strict)"("Visible"=TRUE, "Scale.Maximum"=170.0 ("Scale.Range:Maximum")) -> ()  [unwired: 2 in, 2 out]
            n153 = local write "Test Slider"(w297) -> ()
            n154 = property on="Motor" class="Clust (strict)"("Visible"=w296) -> ()  [unwired: 2 in, 2 out]
            n155 = property on="Rev/Fwd" class="Clust (strict)"("Visible"=w296) -> ()  [unwired: 2 in, 2 out]
            n156 = property on="On/Off" class="Bool (strict)"("Visible"=w296) -> ()  [unwired: 2 in, 2 out]
            n157 = property on="Test Ring" class="Ring (strict)"("Visible"=w296) -> ()  [unwired: 2 in, 2 out]
          }
          frame "Relay", "Solenoid" {
            w299 = FALSE ("Visible")
            n158 = property on="Motor" class="Clust (strict)"("Visible"=w299) -> ()  [unwired: 2 in, 2 out]
            n159 = property on="Test Slider" class="Slide (strict)"("Visible"=w299) -> ()  [unwired: 2 in, 2 out]
            n160 = Search and Replace String(input string=w300, search string="/Value  **", replace string="/Direction") -> (result string=w306:string)  [unwired: 5 in, 3 out]
            n161 = property on="Test Ring" class="Ring (strict)"("Visible"=w299) -> ()  [unwired: 2 in, 2 out]
            n162 = call <vilib>:"NT Read String.vi"("Name"=w306) -> ("String"=w304:string)  [unwired: 9 in, 1 out]
            n163 = Equal?(x="Both directions", y=w304) -> (x = y?=w302:bool)
            n164 = Not(x=w302) -> (.not. x?=w303:bool)
            n165 = property on="Rev/Fwd" class="Clust (strict)"("Visible"=w302) -> ()  [unwired: 2 in, 2 out]
            n166 = property on="On/Off" class="Bool (strict)"("Visible"=w303, "Caption.Text"=w301) -> ()  [unwired: 2 in, 2 out]
          }
          frame "Compressor", "Digital Out" {
            w309 = FALSE ("Visible")
            # "Get direction and finish"
            n167 = property on="Motor" class="Clust (strict)"("Visible"=w309) -> ()  [unwired: 2 in, 2 out]
            n168 = property on="Test Slider" class="Slide (strict)"("Visible"=w309) -> ()  [unwired: 2 in, 2 out]
            n169 = property on="Test Ring" class="Ring (strict)"("Visible"=w309) -> ()  [unwired: 2 in, 2 out]
            n170 = property on="On/Off" class="Bool (strict)"("Visible"=TRUE, "Caption.Text"=w310) -> ()  [unwired: 2 in, 2 out]
            n171 = property on="Rev/Fwd" class="Clust (strict)"("Visible"=FALSE) -> ()  [unwired: 2 in, 2 out]
          }
          frame "Camera" {
            n172 = call <vilib>:"Get Last Path Segment.vi"("String in"=w317) -> ("String out"=w318:string)  [unwired: 10 in]
            n173 = property on="On/Off" class="Bool (strict)"("Visible"=FALSE) -> ()  [unwired: 2 in, 2 out]
            n174 = property on="Motor" class="Clust (strict)"("Visible"=FALSE) -> ()  [unwired: 2 in, 2 out]
            n175 = property on="Rev/Fwd" class="Clust (strict)"("Visible"=FALSE) -> ()  [unwired: 2 in, 2 out]
            n176 = case shown="\"White Balance  **\"" w318 {
              tunnel: w317 -> [w324 w333 w342 w351 w360 _ w366]
              tunnel: w316 -> [w322 w330 w339 w348 w357 _ _]
              frame "Size  **" {
                n177 = Index Array(array=w322) -> (element=w321:cluster{string[]})  [unwired: 1 in]
                n178 = call <vilib>:"NT Read String.vi"("Name"=w324) -> ("String"=w323:string)  [unwired: 9 in, 1 out]
                n179 = Unbundle(w321) -> (w319:string[])
                n180 = Match First String(2:w319, 3:w323) -> (0:w320:i32)  [unwired: 1 out]
                n181 = property on="Test Ring" class="Ring (strict)"("Value"=w320, "Strings []"=w319) -> ()  [unwired: 2 in, 2 out]
                n182 = property on="Test Ring" class="Ring (strict)"("Visible"=TRUE) -> ()  [unwired: 2 in, 2 out]
                n183 = property on="Test Slider" class="Slide (strict)"("Visible"=FALSE) -> ()  [unwired: 2 in, 2 out]
              }
              frame "White Balance  **" {
                n184 = Index Array(array=w330, index=1) -> (element=w331:cluster{string[]})
                n185 = call <vilib>:"NT Read String.vi"("Name"=w333) -> ("String"=w332:string)  [unwired: 9 in, 1 out]
                n186 = Unbundle(w331) -> (w328:string[])
                n187 = Match First String(2:w328, 3:w332) -> (0:w327:i32)  [unwired: 1 out]
                n188 = property on="Test Ring" class="Ring (strict)"("Value"=w327, "Strings []"=w328) -> ()  [unwired: 2 in, 2 out]
                n189 = property on="Test Ring" class="Ring (strict)"("Visible"=TRUE) -> ()  [unwired: 2 in, 2 out]
                n190 = property on="Test Slider" class="Slide (strict)"("Visible"=FALSE) -> ()  [unwired: 2 in, 2 out]
              }
              frame "Exposure  **" {
                n191 = Index Array(array=w339, index=2) -> (element=w340:cluster{string[]})
                n192 = call <vilib>:"NT Read String.vi"("Name"=w342) -> ("String"=w341:string)  [unwired: 9 in, 1 out]
                n193 = Unbundle(w340) -> (w336:string[])
                n194 = Match First String(2:w336, 3:w341) -> (0:w337:i32)  [unwired: 1 out]
                n195 = property on="Test Ring" class="Ring (strict)"("Value"=w337, "Strings []"=w336) -> ()  [unwired: 2 in, 2 out]
                n196 = property on="Test Ring" class="Ring (strict)"("Visible"=TRUE) -> ()  [unwired: 2 in, 2 out]
                n197 = property on="Test Slider" class="Slide (strict)"("Visible"=FALSE) -> ()  [unwired: 2 in, 2 out]
              }
              frame "Exposure Priority  **" {
                n198 = Index Array(array=w348, index=3) -> (element=w349:cluster{string[]})
                n199 = call <vilib>:"NT Read String.vi"("Name"=w351) -> ("String"=w350:string)  [unwired: 9 in, 1 out]
                n200 = Unbundle(w349) -> (w345:string[])
                n201 = Match First String(2:w345, 3:w350) -> (0:w346:i32)  [unwired: 1 out]
                n202 = property on="Test Ring" class="Ring (strict)"("Value"=w346, "Strings []"=w345) -> ()  [unwired: 2 in, 2 out]
                n203 = property on="Test Ring" class="Ring (strict)"("Visible"=TRUE) -> ()  [unwired: 2 in, 2 out]
                n204 = property on="Test Slider" class="Slide (strict)"("Visible"=FALSE) -> ()  [unwired: 2 in, 2 out]
              }
              frame "Color Enable  **" {
                n205 = Index Array(array=w357, index=4) -> (element=w358:cluster{string[]})
                n206 = call <vilib>:"NT Read String.vi"("Name"=w360) -> ("String"=w359:string)  [unwired: 9 in, 1 out]
                n207 = Unbundle(w358) -> (w354:string[])
                n208 = Match First String(2:w354, 3:w359) -> (0:w355:i32)  [unwired: 1 out]
                n209 = property on="Test Ring" class="Ring (strict)"("Value"=w355, "Strings []"=w354) -> ()  [unwired: 2 in, 2 out]
                n210 = property on="Test Ring" class="Ring (strict)"("Visible"=TRUE) -> ()  [unwired: 2 in, 2 out]
                n211 = property on="Test Slider" class="Slide (strict)"("Visible"=FALSE) -> ()  [unwired: 2 in, 2 out]
              }
              frame Default {
                n212 = property on="Test Ring" class="Ring (strict)"("Visible"=FALSE) -> ()  [unwired: 2 in, 2 out]
                n213 = property on="Test Slider" class="Slide (strict)"("Visible"=FALSE) -> ()  [unwired: 2 in, 2 out]
              }
              frame "Brightness  **", "Color Level  **", "Compression  **", "FPS  **", "Sharpness  **" {
                n214 = call <vilib>:"NT Read Number.vi"("Name"=w366) -> ("Numeric"=w365:dbl)  [unwired: 9 in, 1 out]
                n215 = local write "Test Slider"(w365) -> ()
                n216 = property on="Test Slider" class="Slide (strict)"("Visible"=TRUE, "Scale.Maximum"=100.0 ("Scale.Range:Maximum")) -> ()  [unwired: 2 in, 2 out]
                n217 = property on="Test Ring" class="Ring (strict)"("Visible"=FALSE) -> ()  [unwired: 2 in, 2 out]
              }
            }
          }
        }
        n218 = property on="Progress" class="Clust (strict)"("Visible"=FALSE) -> ()  [unwired: 2 in, 2 out]
      }
      event "Test Name": Mouse Enter {
        # "Populate the ring with the list of tests"
        n219 = event-data() -> ()  [unwired: 1 in, 1 out]
        n220 = call <vilib>:"NT Read String Array.vi"("Name"="TestMode/TestList") -> ("String Array"=w374:string[])  [unwired: 9 in, 1 out]
        n221 = Build Array (concatenate)("Select the test to run...", w374) -> (w373:string[])
        n222 = property on="Test Name" class="Ring (strict)"("Strings []"=w373) -> ()  [unwired: 2 in, 2 out]
      }
      event "Test Name": Value Change {
        w376 = FALSE ("Visible")
        # "Tell the robot the test name to run"
        n223 = event-data() -> ("NewVal"=w380:u16)  [unwired: 1 in]
        n224 = property on="Test Name" class="Ring (strict)"() -> ("Strings []"=w381:string[])  [unwired: 2 in, 2 out]
        n225 = local write "Progress"(T6 {"Test Progress"=0, "Test Progress Text"=""} ("Progress")) -> ()
        n226 = Index Array(array=w381, index=w380) -> (element=w379:string)
        n227 = call <vilib>:"NT Write String.vi"("String"=w379, "Name"="TestMode/TestName") -> ()  [unwired: 9 in, 1 out]
        n228 = property on="Progress" class="Clust (strict)"("Visible"=TRUE) -> ()  [unwired: 2 in, 2 out]
        n229 = property on="Motor" class="Clust (strict)"("Visible"=w376) -> ()  [unwired: 2 in, 2 out]
        n230 = property on="Test Slider" class="Slide (strict)"("Visible"=w376) -> ()  [unwired: 2 in, 2 out]
        n231 = property on="On/Off" class="Bool (strict)"("Visible"=w376) -> ()  [unwired: 2 in, 2 out]
        n232 = property on="Rev/Fwd" class="Clust (strict)"("Visible"=w376) -> ()  [unwired: 2 in, 2 out]
        n233 = property on="Test Ring" class="Ring (strict)"("Visible"=w376) -> ()  [unwired: 2 in, 2 out]
      }
      event "Select Auto": Mouse Enter {
        # "Populate the combo box with the list of autonomous options"
        n234 = event-data() -> ()  [unwired: 1 in, 1 out]
        n235 = call <vilib>:"NT Read String Array.vi"("Name"="Auto List") -> ("String Array"=w383:string[])  [unwired: 9 in, 1 out]
        n236 = property on="Select Auto" class="CmbBox"("Strings[]"=w383) -> ()  [unwired: 2 in, 2 out]
      }
      event "Select Auto": Value Change {
        # "User modified the Auto Selection. Write to NT variable so robot knows."
        n237 = event-data() -> ("NewVal"=w386:string)  [unwired: 1 in]
        n238 = call <vilib>:"NT Write String.vi"("String"=w386, "Name"="Auto Selector") -> ()  [unwired: 9 in, 1 out]
      }
      event "Command Selection": Value Change {
        # "Get the params and show in table"
        n239 = event-data() -> ("NewVal"=w392:i32)  [unwired: 1 in]
        n240 = property on="Command Selection" class="MCListbox (strict)"() -> ("ItemNames"=w390:string[][])  [unwired: 2 in, 2 out]
        n241 = call <vilib>:"WPI_DashboardUpdate Command Params.vi"("NewVal"=w392, "Commands"=w390, "Param Tbl"=w391) -> ()  [unwired: 8 in, 1 out]
      }
      event "Execute Command": Value Change {
        # "Started one, Unique ID holds\nresponse"
        n242 = event-data() -> ()  [unwired: 1 in, 1 out]
        n243 = property on="Command Selection" class="MCListbox (strict)"() -> ("ItemNames"=w403:string[][])  [unwired: 2 in, 2 out]
        n244 = Index Array(array=w403, index (row)="Command Selection", index (col)=0) -> (element=w401:string)
        n245 = call <vilib>:"Invoke Commands.vi"("Command Params"="Command Params", "Function Name"=w401) -> ("Params"=w397:u8, "Started"=w396:bool)  [unwired: 7 in, 1 out]
        n246 = Array Subset(array="Command Params", length (row)=w397) -> (w398:string[][])  [unwired: 3 in]
        n247 = Select(t="Executing" ("Cmd Status"), s=w396, f="" ("Cmd Status")) -> (s? t:f=→"Cmd Status":string)
      }
      event "Command Selection": Double Click {
        n248 = event-data() -> ("Row"=w411:i32)  [unwired: 1 in]
        n249 = property on="Command Selection" class="MCListbox (strict)"() -> ("ItemNames"=w414:string[][])  [unwired: 2 in, 2 out]
        n250 = local read "Command Params"() -> (w410:string[][])
        n251 = Index Array(array=w414, index (row)=w411, index (col)=0) -> (element=w412:string)
        n252 = call <vilib>:"Invoke Commands.vi"("Command Params"=w410, "Function Name"=w412) -> ("Params"=w409:u8, "Started"=w404:bool)  [unwired: 7 in, 1 out]
        n253 = Array Subset(array=w410, length (row)=w409) -> (w408:string[][])  [unwired: 3 in]
        n254 = Select(t="Executing" ("Cmd Status"), s=w404, f="" ("Cmd Status")) -> (s? t:f=w405:string)
        n255 = local write "Cmd Status"(w405) -> ()
      }
      event "CheckList": Double Click {
        # "Shift clears all"
        # "Update symbols on the listbox"
        n256 = event-data() -> ("PlatMods.Shift"=w416:bool, "Row"=w418:i32)  [unwired: 1 in]
        n257 = case shown="True" w416 {
          tunnel: w418 -> [w422 _]
          tunnel: 1 -> [w421 _]
          frame False {
            n258 = property on="CheckList" class="LstBox (strict)"() -> ("Item Symbols"=w420:i32[])  [unwired: 2 in, 2 out]
            n259 = Replace Array Subset(array=w420, new element=w421, index=w422) -> (w419:i32[])
            n260 = property on="CheckList" class="LstBox (strict)"("Item Symbols"=w419) -> ()  [unwired: 2 in, 2 out]
          }
          frame True {
            w423 = 0 ("Top Row")
            n261 = property on="CheckList" class="LstBox (strict)"() -> ("Number of Rows"=w425:u32)  [unwired: 2 in, 2 out]
            n262 = Initialize Array(0, w425) -> (w424:i32[])
            n263 = property on="CheckList" class="LstBox (strict)"("Top Row"=w423, "Value"=w423, "Item Symbols"=w424) -> ()  [unwired: 2 in, 2 out]
          }
        }
      }
      event "CheckList": Key Down {
        # "Update symbols on the listbox\nLeft and right keys check and uncheck"
        n264 = event-data() -> ("VKey"=w429:T24)  [unwired: 1 in]
        n265 = case shown="\"Left\", \"Right\"" w429 {
          selector: w429 -> [w434 _]
          tunnel: eventvkey."Left" ("VKey") -> [w432 _]
          frame "Left", "Right" {
            n266 = Equal?(x=w432, y=w434) -> (x = y?=w433:bool)
            n267 = Select(t=0, s=w433, f=1) -> (s? t:f=w435:i32)
            n268 = property on="CheckList" class="LstBox (strict)"() -> ("Item Symbols"=w438:i32[])  [unwired: 2 in, 2 out]
            n269 = Replace Array Subset(array=w438, new element=w435, index="CheckList") -> (w437:i32[])
            n270 = property on="CheckList" class="LstBox (strict)"("Item Symbols"=w437) -> ()  [unwired: 2 in, 2 out]
          }
          frame Default {
          }
        }
      }
      event "Motor.Enable": Value Change {
        # "When the test mode otor enable helper is set, update that\ntree row item's value"
        n271 = event-data() -> ("NewVal"=w444:bool)  [unwired: 1 in]
        n272 = Unbundle("Motor") -> ("Value"=w443:dbl)  [unwired: 1 out]
        n273 = Select(t=w443, s=w444, f=0.0) -> (s? t:f=w441:dbl)
        n274 = call <vilib>:"NT Write Number.vi"("Numeric"=w441, "Name"=w440) -> ()  [unwired: 9 in, 1 out]
      }
      event "Test Slider": Value Change {
        # "When the test mode slider helper is set, update that\ntree row item's value"
        n275 = event-data() -> ("NewVal"=w447:dbl)  [unwired: 1 in]
        n276 = call <vilib>:"NT Write Number.vi"("Numeric"=w447, "Name"=w448) -> ()  [unwired: 9 in, 1 out]
      }
      event "On/Off": Value Change {
        # "When the test mode on/off helper value is set, update that\ntree row item's value"
        n277 = event-data() -> ("NewVal"=w452:bool)  [unwired: 1 in]
        n278 = Boolean To (0,1)(Boolean=w452) -> (0, 1=w451:i16)
        n279 = call <vilib>:"NT Write Number.vi"("Numeric"=w451, "Name"=w450) -> ()  [unwired: 9 in, 1 out]
      }
      event "Rev/Fwd": Value Change {
        # "When the test mode helper value for relays is set, update that\ntree row item's value"
        n280 = event-data() -> ("NewVal.Forward"=w460:bool, "NewVal.Reverse"=w459:bool)  [unwired: 1 in]
        n281 = Boolean To (0,1)(Boolean=w460) -> (0, 1=w456:i16)
        n282 = Boolean To (0,1)(Boolean=w459) -> (0, 1=w458:i16)
        n283 = Negate(x=w458) -> (-x=w457:i16)
        n284 = Add(x=w456, y=w457) -> (x+y=w455:i16)
        n285 = call <vilib>:"NT Write Number.vi"("Numeric"=w455, "Name"=w454) -> ()  [unwired: 9 in, 1 out]
      }
      event "Test Ring": Value Change {
        # "When a test mode helper value is selected from the ring,\nset the tree item's variable to the string value"
        n286 = event-data() -> ("NewVal"=w464:u16)  [unwired: 1 in]
        n287 = property on="Test Ring" class="Ring (strict)"() -> ("Strings []"=w465:string[])  [unwired: 2 in, 2 out]
        n288 = Index Array(array=w465, index=w464) -> (element=w463:string)
        n289 = call <vilib>:"NT Write String.vi"("String"=w463, "Name"=w462) -> ()  [unwired: 9 in, 1 out]
      }
      event "Rec Mode": Value Change {
        # "Update globals for recording mode and path to read log from.\nClear when logging and let NetworkTables set path for vision to\nuse."
        n290 = event-data() -> ("NewVal"=w476:enum32{"Stop", "Record", "Playback"})  [unwired: 1 in]
        n291 = global write "WPI_DashboardLogging Global.vi" "Logging Filename"(path "") -> ()
        n292 = global write "WPI_DashboardLogging Global.vi" "Recording"(w476) -> ()
        n293 = case shown="\"Playback\"" w476 {
          tunnel: w475 -> [_ w478 w487]
          tunnel: [_ _ w486] -> w473
          tunnel: [_ _ w485] -> _
          tunnel: w471 -> [_ _ w483]
          tunnel: cluster{i32, i32} {-250, 170} -> [_ _ w482]
          tunnel: [_ _ T25 {"Image Size"=TRUE, "Image Type"=TRUE, "Pixel Value"=TRUE, "ROI Information"=TRUE, "Zoom Factor"=FALSE} ("Image Information Shown:All Elements")] -> w466
          tunnel: [_ _ TRUE ("Zoom Factor")] -> w467
          tunnel: w469 -> [_ _ w479]
          frame Default {
          }
          frame "Stop", "Record" {
            # "Place Window too"
            n294 = invoke class="VI" method="FP.Close"(reference=w478) -> (reference out=w477:refnum<vi>)  [unwired: 2 in, 2 out]
            n295 = invoke class="VI" method="Abort VI"(reference=w477) -> ()  [unwired: 2 in, 3 out]
          }
          frame "Playback" {
            n296 = call "Open Playback Panel.vi"("Offset"=w482, "DB VI Ref"=w483, "Playback in"=w487) -> ("Playback out"=w484:refnum<vi>)  [unwired: 8 in]
            n297 = register-events(w484, w479) -> (reference out=w486:refnum<event-registration>, error out=w485:errorcluster)  [unwired: 2 in]
          }
        }
        n298 = property on="Camera Image Right" class="ImageControl"("Image Information Shown"=w466, "Image Information Visible"=w467) -> ()  [unwired: 2 in, 2 out]
        n299 = property on="Camera Image" class="ImageControl"("Image Information Shown"=w466, "Image Information Visible"=w467) -> ()  [unwired: 2 in, 2 out]
        n300 = call <vilib>:"WPI_DashboardNT Log FieldName Cache.vi"("Operation"=enum16{"Lookup/Add", "Index", "Clear"}."Clear") -> ()  [unwired: 8 in, 3 out]
      }
      event Panel Close {
        w489 = enum32{"Stop", "Record", "Playback"}."Stop" ("Rec Mode")
        # "Playback window has been closed, abort"
        n301 = event-data() -> ()  [unwired: 1 in, 4 out]
        n302 = local write "Rec Mode"(w489) -> ()
        n303 = global write "WPI_DashboardLogging Global.vi" "Recording"(w489) -> ()
      }
      event Panel Close {
        # "Abort playback window and ourself"
        n304 = event-data() -> ()  [unwired: 1 in, 4 out]
        n305 = invoke class="VI" method="FP.Close"(reference=w493) -> (reference out=w492:refnum<vi>)  [unwired: 2 in, 2 out]
        n306 = invoke class="VI" method="Abort VI"(reference=w492) -> (error out=w491:errorcluster)  [unwired: 2 in, 2 out]
        n307 = invoke class="VI" method="Abort VI"(error in=w491) -> ()  [unwired: 2 in, 3 out]
      }
      event User Event {
        n308 = event-data() -> ("IDs"=w500:cluster{"RPC field ID":u16, "Unique ID":u16}, "String"=w499:string)  [unwired: 1 in]
        n309 = Bundle("IDs"=w500, "String"=w499) -> (w498:T9)  [unwired: 1 in]
        n310 = call <vilib>:"Retrieve RPC Response.vi"("RPC Response"=w498) -> ("Output"=w496:string[][])  [unwired: 10 in]
        n311 = Build Array (concatenate)(w494, w496) -> (w495:string[][])
        n312 = local write "Command Params"(w495) -> ()
        n313 = local write "Cmd Status"("" ("Cmd Status")) -> ()
      }
      event "Tree": Double Click {
        n314 = event-data() -> ("PlatMods"=w506:T28, "Tag"=w503:string)  [unwired: 1 in]
        n315 = Unbundle(w506) -> ("Shift"=w505:bool)  [unwired: 4 out]
        n316 = String Subset(string=w503, length (rest)=1 ("length (rest)")) -> (substring=w502:string)  [unwired: 1 in]
        n317 = Not(x=w505) -> (.not. x?=w504:bool)
        n318 = case shown="\"/\"" w502 {
          tunnel: w503 -> [_ w509]
          tunnel: w504 -> [_ w508]
          frame Default {
          }
          frame "/" {
            n319 = call <vilib>:"NT Update Persistence.vi"("Persistence"=w508, "Name"=w509) -> ()  [unwired: 9 in, 1 out]
          }
        }
      }
    }
  }
  n320 = while {
    tunnel: w66 -> [w511]
    i -> [w514]
    stop <- FALSE stop-if-true
    n321 = Wait (ms)(milliseconds to wait=u32 100) -> ()  [unwired: 1 out]
    n322 = case shown="\"Playback\"" "Rec Mode" {
      tunnel: w514 -> [_ _ w529]
      tunnel: [u32 2829099 ("Base Color") u32 11141120 ("Target Color") w518] -> w510
      frame "Stop", Default {
        # "Reset the color, extra updates don't cost much"
      }
      frame "Record" {
      }
      frame "Playback" {
        # "Playback"
        n323 = Quotient & Remainder(x=w529, y=u32 50 ("milliseconds to wait")) -> (x-y*floor(x/y)=w525:u32)  [unwired: 1 out]
        n324 = Divide(x=w525, y=u32 50 ("milliseconds to wait")) -> (x/y=w522:dbl)
        n325 = Multiply(x=6.283185307179586, y=w522) -> (x*y=w527:dbl)
        n326 = Sine(x=w527) -> (sin(x)=w526:dbl)
        n327 = Absolute Value(x=w526) -> (abs(x)=w519:dbl)
        n328 = call "Interpolate RGB Color.vi"("Proportion"=w519, "Target Color"=u32 30976, "Base Color"=u32 2829099) -> ("Result Color"=w518:u32)  [unwired: 8 in]
      }
    }
    n329 = property class="Pane"(reference=w511, "PaneColor"=w510) -> ()  [unwired: 1 in, 2 out]
  }
  n330 = local write "Dashboard Tab"(T2."Drive" ("Dashboard Tab")) -> ()
  n331 = property on="On/Off" class="Bool (strict)"("Visible"=w37) -> ()  [unwired: 2 in, 2 out]
  n332 = property on="Motor" class="Clust (strict)"("Visible"=w37) -> ()  [unwired: 2 in, 2 out]
  n333 = property on="Progress" class="Clust (strict)"("Visible"=w37) -> ()  [unwired: 2 in, 2 out]
  n334 = property on="Test Ring" class="Ring (strict)"("Visible"=w37) -> ()  [unwired: 2 in, 2 out]
  n335 = property on="Rev/Fwd" class="Clust (strict)"("Visible"=w37) -> ()  [unwired: 2 in, 2 out]
  n336 = while {
    tunnel: u16 1741 ("timeout ms (25000)") -> [w531]
    stop <- FALSE stop-if-true
    n337 = TCP Create Listener(10:w531) -> (0:w530:errorcluster, 3:w532:refnum<k5>)  [unwired: 4 in, 1 out]
    n338 = case shown="No Error" w530 {
      selector: w530 -> [w534 _]
      tunnel: w532 -> [w535 _]
      frame No Error {
        n339 = while {
          tunnel: w535 -> [w538]
          tunnel: w534 -> [w537]
          stop <- FALSE stop-if-true
          n340 = TCP Wait On Listener(8:w537, 11:w538) -> (0:w539:errorcluster, 4:w540:refnum<k5>)  [unwired: 2 in, 3 out]
          n341 = local write "TCP"(w540) -> ()
          n342 = case shown="No Error" w539 {
            frame No Error {
            }
            frame Error {
              n343 = Wait (ms)(milliseconds to wait=u32 1000) -> ()  [unwired: 1 out]
            }
          }
        }
      }
      frame Error {
        n344 = Wait (ms)(milliseconds to wait=u32 1000) -> ()  [unwired: 1 out]
      }
    }
  }
  n345 = local write "Command Selection"(u16 0 ("milliseconds to wait")) -> ()
  n346 = local write "Command Params"(string[][] [] ("Command Params")) -> ()
  n347 = global write "WPI_DashboardLogging Global.vi" "Recording"(w60) -> ()
  n348 = local write "Rec Mode"(w60) -> ()
  n349 = call <vilib>:"NT Write String.vi"("String"="Select Auto", "Name"="Auto Selector") -> ()  [unwired: 9 in, 1 out]
